vi "FGV測試.vi"() -> ()   [LabVIEW 2015]
uses:
  <userlib>/FGV/control/Control_Image.ctl
  <userlib>/FGV/control/Control_Camera.ctl
panel:
  in  "開檔":bool=TRUE
  in  "error in (no error)":errorcluster
  out "error out":errorcluster
  out "Image":T1(plugin-control)
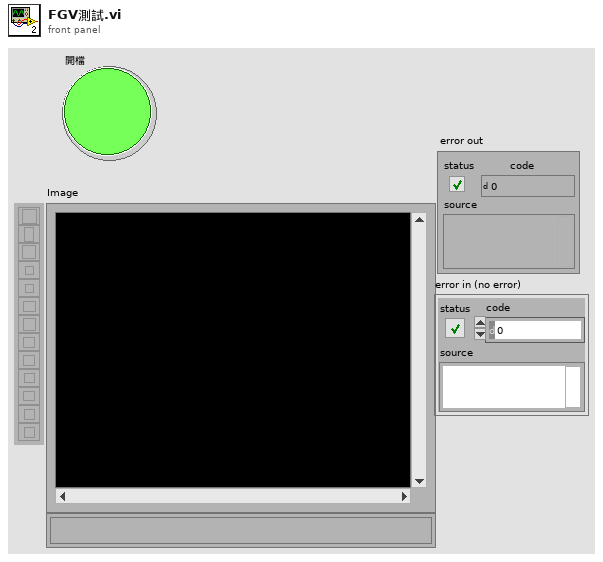
[diagram p1: front panel]
types:
  T1 = typedef "IMAQ Image.ctl" = refnum<image>
  T2 = typedef "Control_Image.ctl" = enum16{"初始化", "創造記憶體", "寫入圖片", "讀取圖片", "刪除圖片", "等待"}
  T3 = typedef "IMAQdx.ctl" = refnum<k21>
  T4 = typedef "Control_Camera.ctl" = enum16{"初始化", "取像", "匯入影像", "結束"}
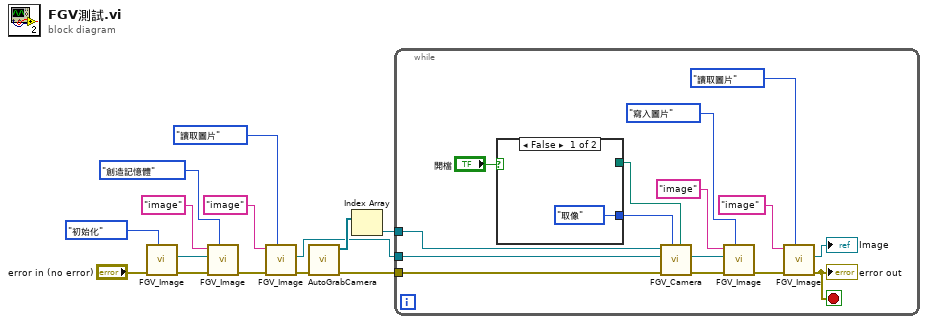
[diagram p0: block diagram]
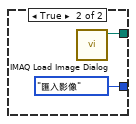
[diagram p2: hidden frame]
diagram:
  n1 = call <userlib>:"FGV_Image.vi"("Image action"=Control_Image."初始化", "error in (no error)"="error in (no error)") -> ("error out"=w7:errorcluster, "Image Out"=w8:T1)  [unwired: 8 in]
  n2 = call <userlib>:"FGV_Image.vi"("Image action"=Control_Image."創造記憶體", "error in (no error)"=w7, "Image In"=w8, "圖片名稱"="image") -> ("error out"=w6:errorcluster)  [unwired: 6 in, 1 out]
  n3 = call <userlib>:"FGV_Image.vi"("Image action"=Control_Image."讀取圖片", "error in (no error)"=w6, "圖片名稱"="image") -> ("error out"=w5:errorcluster, "Image Out"=w2:T1)  [unwired: 7 in]
  n4 = call <userlib>:"AutoGrabCamera.vi"("error in"=w5) -> ("error out"=w1:errorcluster, "Session Out Array"=w14:T3[])  [unwired: 9 in]
  n5 = Index Array(array=w14) -> (element=w3:T3)  [unwired: 1 in]
  n6 = while {
    tunnel: w3 -> [w29]
    tunnel: w2 -> [w28]
    tunnel: w1 -> [w27]
    stop <- w16 stop-if-true
    n7 = case shown="False" "開檔" {
      tunnel: [Control_Camera."取像" ("action_camera") Control_Camera."匯入影像" ("action_camera")] -> w18
      tunnel: [_ w31] -> w17
      frame False {
      }
      frame True {
        n8 = call "IMAQ Load Image Dialog"() -> ("Path"=w31:path)  [unwired: 9 in, 2 out]
      }
    }
    n9 = call <userlib>:"FGV_Camera.vi"("File Path"=w17, "action_camera"=w18, "error in"=w27, "Image In"=w28, "Session In"=w29) -> ("error out"=w20:errorcluster, "Image Out"=w26:T1)  [unwired: 4 in, 1 out]
    n10 = call <userlib>:"FGV_Image.vi"("Image action"=Control_Image."寫入圖片", "error in (no error)"=w20, "Image In"=w26, "圖片名稱"="image") -> ("error out"=w21:errorcluster)  [unwired: 6 in, 1 out]
    n11 = call <userlib>:"FGV_Image.vi"("Image action"=Control_Image."讀取圖片", "error in (no error)"=w21, "圖片名稱"="image") -> ("error out"=w16:errorcluster, "Image Out"=→"Image":T1)  [unwired: 7 in]
    "error out" <- w16
  }
